vi "Network Command Engine.vi"(8 "error in (no error)":errorcluster, 11 "State Variables":T1={"TCP Refs"={"Connection List"=refnum, "listener ID"=refnum}, "Stop"=refnum, "Top VI"=refnum, "Parameters"={"Name"="", "PID Lookup"=variant, "DID Lookup"=variant, "Section Properties"={"CAN"={"Database File"=path "", "CAN Interface"=enum."CAN0", "Baud Rate"=0, "Diagnostic Protocol"=enum."GMLAN", "Transport Protocol"=enum."ISO TP - Normal Mode", "Transmit ID"=0, "Receive ID"=0, "Transmit Extension"=0, "Receive Extension"=0, "Receive UUDT ID"=0, "Enable Stream"=TRUE, "VW TP Channel ID"=0}, "DPIDs"=[], "DTC descriptor"={"DTC Byte Length"=2, "Status Byte Length"=1, "Add Data Byte Length"=1, "Byte Order"=enum."Motorola"}, "PIDs"=[], "DIDs"=[], "CPIDs"=[]}, "ChanRefs"={"ToVS.PIDs"={"Name"="", "Write to VS Engine FIFO"=refnum, "Pairs"={"Refs"=[], "Values"=[]}}, "ToVS.DIDs"={"Name"="", "Write to VS Engine FIFO"=refnum, "Pairs"={"Refs"=[], "Values"=[]}}, "ToVS.DTCs"={"Name"="", "Write to VS Engine FIFO"=refnum, "Pairs"={"Refs"=[], "Values"=[]}}, "ToVS.DTCCount"={"Name"="", "Write to VS Engine FIFO"=refnum, "Pairs"={"Refs"=[], "Values"=[]}}, "ToVS.Success"={"Name"="", "Write to VS Engine FIFO"=refnum, "Pairs"={"Refs"=[], "Values"=[]}}, "FromVS.CPIDs"={"Name"="", "Read from VS Engine FIFO"=refnum, "Pairs"={"Refs"=[], "Values"=[]}}, "Cmds"={"Name"="", "Write to VS Engine FIFO"=refnum, "Read from VS Engine FIFO"=refnum, "Pairs"={"Chan Refs"=[], "Prev. Values"=[]}}}, "CPID Lookup"=variant, "DPID Lookup"=variant}, "ADCS Connection"={"Diag CAN Handle"=0, "Transport Protocol"=enum."ISO TP - Normal Mode", "Receive Address Extension"=0, "Transmit Address Extension"=0, "Receive CAN Id"=0, "Transmit CAN Id"=0, "Diag CAN Queue"=refnum, "Log Frames ?"=FALSE, "My TP Address"=0, "Other TP Address"=0, "T1"=0, "T2"=0, "T3"=0, "T4"=0, "Tx SN"=0, "Block Size"=0, "Rx SN"=0, "VW TP Initialized?"=FALSE, "Tx block no"=0, "baud rate"=0, "Interface"="", "Channel Diag CAN Handle"=0, "UDP Connection ID"=refnum, "TCP Connection ID"=refnum, "Target IP Addr"=0, "Source Address"=0, "Target Address"=0, "Send Header NACK?"=FALSE, "DLL Handle"=0, "NAD"=0, "Time Stamp read first"=0.0, "Time Stamp read last"=0.0, "Time Stamp write first"=0.0, "Time Stamp write last"=0.0, "Time Stamp write"=0.0, "Time Stamp read"=0.0}, "XNET References"={"Database"="", "GMLAN DPID Session"="", "Cluster"=""}, "BufferedCmds"=refnum, "XNETEngine (GMLAN)"=refnum} {"Parameters"."ChanRefs"."Cmds"."Pairs"."Chan Refs" format="%.0x"; "Parameters"."ChanRefs"."ToVS.Success"."Pairs"."Refs" format="%.0x"; "Parameters"."ChanRefs"."ToVS.DTCCount"."Pairs"."Refs" format="%.0x"; "Parameters"."ChanRefs"."ToVS.DTCs"."Pairs"."Refs" format="%.0x"; "Parameters"."ChanRefs"."ToVS.PIDs"."Pairs"."Refs" format="%.0x"; "Parameters"."ChanRefs"."ToVS.DIDs"."Pairs"."Refs" format="%.0x"; "Parameters"."Section Properties"."CPIDs"."Signals"."Byte Order" items=["Little Endian", "Big Endian"]; "Parameters"."Section Properties"."CPIDs"."Signals"."Data Type" items=["Signed", "Unsigned", "IEEE Float"]; "Parameters"."Section Properties"."DIDs"."Signals"."Byte Order" items=["Little Endian", "Big Endian"]; "Parameters"."Section Properties"."DIDs"."Signals"."Data Type" items=["Signed", "Unsigned", "IEEE Float"]; "Parameters"."Section Properties"."CAN"."VW TP Channel ID" format="%.0x"; "Parameters"."Section Properties"."CAN"."Receive UUDT ID" format="%.0x"; "Parameters"."Section Properties"."CAN"."Receive Extension" format="%.0x"; "Parameters"."Section Properties"."CAN"."Transmit Extension" format="%.0x"; "Parameters"."Section Properties"."CAN"."Receive ID" format="%.0x"; "Parameters"."Section Properties"."CAN"."Transmit ID" format="%.0x"; "Parameters"."Section Properties"."PIDs"."Signals"."Byte Order" items=["Little Endian", "Big Endian"]; "Parameters"."Section Properties"."PIDs"."Signals"."Data Type" items=["Signed", "Unsigned", "IEEE Float"]}) -> (0 "error out":errorcluster)   [LabVIEW 2015, in "Diagnostics Addon Engine.lvlib"]
uses:
  Diagnostics Addon Engine.lvlib
  State Variables.ctl
  TCP Refs.ctl
  STM/STM Lookup Table Ref.ctl
  Stop FG/Stop Global Ref.ctl
  Main Configuration.ctl
  Section Properties.ctl
  Shared/CAN Configuration.ctl
  Shared/CAN Interface.ctl
  Shared/Diagnostic Protocols.ctl
  Shared/Transport Protocols.ctl
  Shared/DPID Parameters.ctl
  Shared/DPID Periodic Rate.ctl
  <vilib>/Automotive Diagnostic Command Set/Diagnostic Protocols.llb/DTC Descriptor.ctl
  Shared/DIDPID Parameters.ctl
  Shared/DIDPID Signal Parameters.ctl
  VS Data Channels.ctl
  Inline Async API/Controls/Write To VS Engine.ctl
  <vilib>/NI Veristand/Custom Device API/Data Reference.ctl
  Inline Async API/Controls/Read From VS Engine.ctl
  <vilib>/NI Veristand/Custom Device API/Block Data Reference.ctl
  Inline Async API/Controls/ReadWrite Data.ctl
  <vilib>/Automotive Diagnostic Command Set/Diagnostic Transport.llb/Diag Reference.ctl
  <vilib>/Automotive Diagnostic Command Set/Diagnostic Transport.llb/Transport Protocol Selector.ctl
  <vilib>/Automotive Diagnostic Command Set/Diagnostic Transport.llb/Diag CAN Frame Log.ctl
  XNET References.ctl
  <vilib>/NI/AMC/Message Queue.ctl
  <vilib>/NI/AMC/Message.ctl
  <vilib>/NI/Tools/Keyed Array/KeyedArray.ctl
  STM/Connection Manager/stm_TCPConnectionMethod.ctl
  Stop FG/Stop Global Commands.ctl
  STM/TCP/stm_TCP Read Options.ctl
  Shared/RequestResponse Data Cluster.ctl
  STM/TCP/stm_TCP Write Options.ctl
  STM/_SubVIs/stm_MetaDataElement.ctl
  <vilib>/NI/Tools/Keyed Array/Map String.vi
  <vilib>/NI/AMC/Create Single Message.vi
  <vilib>/NI/AMC/Update Message Routing Info.vi
  <vilib>/NI/AMC/Read Termination Message.vi
  <vilib>/NI/Tools/String/Get Case Matching.vi
  <vilib>/NI/AMC/Send Message.vi
  <vilib>/NI/AMC/Globals.vi
  Shared/GUID Lookup.vi
  Stop FG/Stop FG.lvlib
  Error Handling API/Error Handling API.lvlib
  Shared/Diagnostics Addon Shared.lvlib
  <vilib>/NI Veristand/Custom Device Tools/Custom Device Utility Library/Custom Device Utility Library.lvlib
  <vilib>/NI/Tools/Keyed Array/Tools_KeyedArray.lvlib
  <vilib>/NI/AMC/AMC.lvlib
  <vilib>/NI Veristand/Custom Device API/Custom Device API.lvlib
  <vilib>/addons/Automotive Diagnostic Command Set/NI_Automotive Diagnostic Command Set.lvlib
  Inline Async API/Inline Async API.lvlib
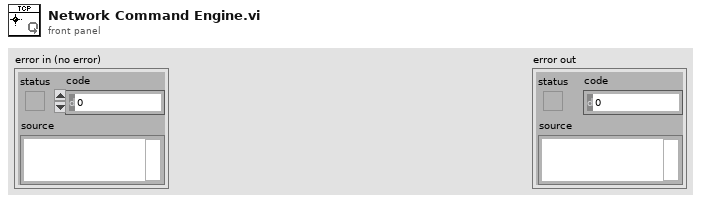
[diagram p1: front panel]
types:
  T1 = typedef "Diagnostics Addon Engine.lvlib/State Variables.ctl" = cluster{"TCP Refs":T2, "Stop":T4, "Top VI":refnum<vi>, "Parameters":T5, "ADCS Connection":T22, "XNET References":T24, "BufferedCmds":T25, "XNETEngine (GMLAN)":T25}
  T2 = typedef "Diagnostics Addon Engine.lvlib/TCP Refs.ctl" = cluster{"Connection List":T3, "listener ID":refnum<k5>}
  T3 = typedef "Diagnostics Addon Engine.lvlib/STM Lookup Table Ref.ctl" = refnum<vi>
  T4 = typedef "Diagnostics Addon Engine.lvlib/Stop FG.lvlib/Stop Global Ref.ctl" = refnum<vi>
  T5 = typedef "Diagnostics Addon Engine.lvlib/Main Configuration.ctl" = cluster{"Name":string, "PID Lookup":variant, "DID Lookup":variant, "Section Properties":T6, "ChanRefs":T16, "CPID Lookup":variant, "DPID Lookup":variant}
  T6 = typedef "Diagnostics Addon Engine.lvlib/Section Properties.ctl" = cluster{"CAN":T7, "DPIDs":T11[], "DTC descriptor":T13, "PIDs":T14[], "DIDs":T14[], "CPIDs":T14[]}
  T7 = typedef "Diagnostics Addon Shared.lvlib/CAN Configuration.ctl" = cluster{"Database File":path, "CAN Interface":T8, "Baud Rate":u32, "Diagnostic Protocol":T9, "Transport Protocol":T10, "Transmit ID":u32, "Receive ID":u32, "Transmit Extension":u8, "Receive Extension":u8, "Receive UUDT ID":u32, "Enable Stream":bool, "VW TP Channel ID":u32}
  T8 = typedef "Diagnostics Addon Shared.lvlib/CAN Interface.ctl" = enum16{"CAN0", "CAN1", "CAN2", "CAN3", "CAN4", "CAN5", "CAN6", "CAN7", "CAN8", "CAN9", "CAN10", "CAN11", "CAN12", "CAN13", "CAN14", "CAN15", "CAN16", "CAN17", "CAN18", "CAN19", "CAN20", "CAN21", "CAN22", "CAN23", "CAN24", "CAN25", "CAN26", "CAN27", "CAN28", "CAN29", "CAN30", "CAN31", "CAN32", "CAN33", "CAN34", "CAN35", "CAN36", "CAN37", "CAN38", "CAN39", "CAN40", "CAN41", "CAN42", "CAN43", "CAN44", "CAN45", "CAN46", "CAN47", "CAN48", "CAN49", "CAN50", "CAN51", "CAN52", "CAN53", "CAN54", "CAN55", "CAN56", "CAN57", "CAN58", "CAN59", "CAN60", "CAN61", "CAN62", "CAN63", "CAN 256 (Virtual)", "CAN 257 (Virtual)"}
  T9 = typedef "Diagnostics Addon Shared.lvlib/Diagnostic Protocols.ctl" = enum16{"GMLAN", "KWP-2000", "UDS"}
  T10 = typedef "Diagnostics Addon Shared.lvlib/Transport Protocols.ctl" = enum16{"ISO TP - Normal Mode", "ISO TP - Mixed Mode", "VW TP 2.0", "Diagnostics on IP"}
  T11 = typedef "Diagnostics Addon Shared.lvlib/DPID Parameters.ctl" = cluster{"DPID ID":u8, "Speed":T12, "PIDs":u16[]}
  T12 = typedef "Diagnostics Addon Shared.lvlib/DPID Periodic Rate.ctl" = enum16{"Slow", "Medium", "Fast"}
  T13 = typedef "DTC Descriptor.ctl" = cluster{"DTC Byte Length":i32, "Status Byte Length":i32, "Add Data Byte Length":i32, "Byte Order":enum16{"Motorola", "Intel"}}
  T14 = typedef "Diagnostics Addon Shared.lvlib/DIDPID Parameters.ctl" = cluster{"Name":string, "Description":string, "ID":u16, "Signals":T15[]}
  T15 = typedef "Diagnostics Addon Shared.lvlib/DIDPID Signal Parameters.ctl" = cluster{"Start Bit":u8, "Length":u8, "Scaling Factor":dbl, "Scaling Offset":dbl, "Minimum":dbl, "Maximum":dbl, "Data Type":u32, "Byte Order":u32, "Default Value":dbl, "Name":string, "Units":string, "Description":string}
  T16 = typedef "Diagnostics Addon Engine.lvlib/VS Data Channels.ctl" = cluster{"ToVS.PIDs":T17, "ToVS.DIDs":T17, "ToVS.DTCs":T17, "ToVS.DTCCount":T17, "ToVS.Success":T17, "FromVS.CPIDs":T19, "Cmds":T21}
  T17 = typedef "Diagnostics Addon Engine.lvlib/Inline Async API.lvlib/Write To VS Engine.ctl" = cluster{"Name":string, "Write to VS Engine FIFO":refnum<k33>, "Pairs":cluster{"Refs":T18[], "Values":dbl[]}}
  T18 = typedef "Custom Device API.lvlib/Data Reference.ctl" = i32
  T19 = typedef "Diagnostics Addon Engine.lvlib/Inline Async API.lvlib/Read From VS Engine.ctl" = cluster{"Name":string, "Read from VS Engine FIFO":refnum<k33>, "Pairs":cluster{"Refs":T20[], "Values":dbl[]}}
  T20 = typedef "Custom Device API.lvlib/Block Data Reference.ctl" = cluster{"Data Reference":T18, "Offset":u64, "Length":u64}
  T21 = typedef "Diagnostics Addon Engine.lvlib/Inline Async API.lvlib/ReadWrite Data.ctl" = cluster{"Name":string, "Write to VS Engine FIFO":refnum<k33>, "Read from VS Engine FIFO":refnum<k33>, "Pairs":cluster{"Chan Refs":T18[], "Prev. Values":dbl[]}}
  T22 = typedef "NI_Automotive Diagnostic Command Set.lvlib/Diag Reference.ctl" = cluster{"Diag CAN Handle":u32, "Transport Protocol":T23, "Receive Address Extension":u8, "Transmit Address Extension":u8, "Receive CAN Id":u32, "Transmit CAN Id":u32, "Diag CAN Queue":refnum<queue>, "Log Frames ?":bool, "My TP Address":u8, "Other TP Address":u8, "T1":u16, "T2":u16, "T3":u16, "T4":u16, "Tx SN":u8, "Block Size":u8, "Rx SN":u8, "VW TP Initialized?":bool, "Tx block no":u8, "baud rate":u32, "Interface":string, "Channel Diag CAN Handle":u32, "UDP Connection ID":refnum<k16>, "TCP Connection ID":refnum<k5>, "Target IP Addr":u32, "Source Address":u16, "Target Address":u16, "Send Header NACK?":bool, "DLL Handle":u32, "NAD":u8, "Time Stamp read first":dbl, "Time Stamp read last":dbl, "Time Stamp write first":dbl, "Time Stamp write last":dbl, "Time Stamp write":dbl, "Time Stamp read":dbl}
  T23 = typedef "NI_Automotive Diagnostic Command Set.lvlib/Transport Protocol Selector.ctl" = enum16{"ISO TP - Normal Mode", "ISO TP - Mixed Mode", "VW TP 2.0", "Diagnostics on IP", "ISO TP LIN"}
  T24 = typedef "Diagnostics Addon Engine.lvlib/XNET References.ctl" = cluster{"Database":refnum<k21>, "GMLAN DPID Session":refnum<k21>, "Cluster":refnum<k21>}
  T25 = typedef "AMC.lvlib/Message Queue.ctl" = refnum<queue>
  T26 = typedef "Diagnostics Addon Engine.lvlib/Stop FG.lvlib/Stop Global Commands.ctl" = enum16{"Write", "Read", "Reset"}
  T27 = typedef "Diagnostics Addon Engine.lvlib/stm_TCPConnectionMethod.ctl" = enum16{"Initialize", "Add Connection", "Set Properties", "Get Connection(s)", "Remove Connection", "Remove All Connections", "Get Connection Count"}
  T28 = typedef "Diagnostics Addon Engine.lvlib/stm_TCP Read Options.ctl" = cluster{"Ignore Timeout Error":bool, "timeout ms (1000)":i32}
  T29 = typedef "Diagnostics Addon Engine.lvlib/stm_TCP Write Options.ctl" = cluster{"Ignore Timeout Error":bool, "timeout ms (1000)":i32}
  T30 = typedef "Diagnostics Addon Shared.lvlib/RequestResponse Data Cluster.ctl" = cluster{"Timeout":i32, "data":string}
  T31 = typedef "Diagnostics Addon Engine.lvlib/stm_MetaDataElement.ctl" = string
  T32 = typedef "Diagnostics Addon Engine.lvlib/stm_TCP Connection Info.ctl" = cluster{"connection ID":refnum<k5>, "Meta data":T31[]}
  T33 = typedef "Tools_KeyedArray.lvlib/KeyedArray.ctl" = cluster{"keys":string[], "values":string[]}
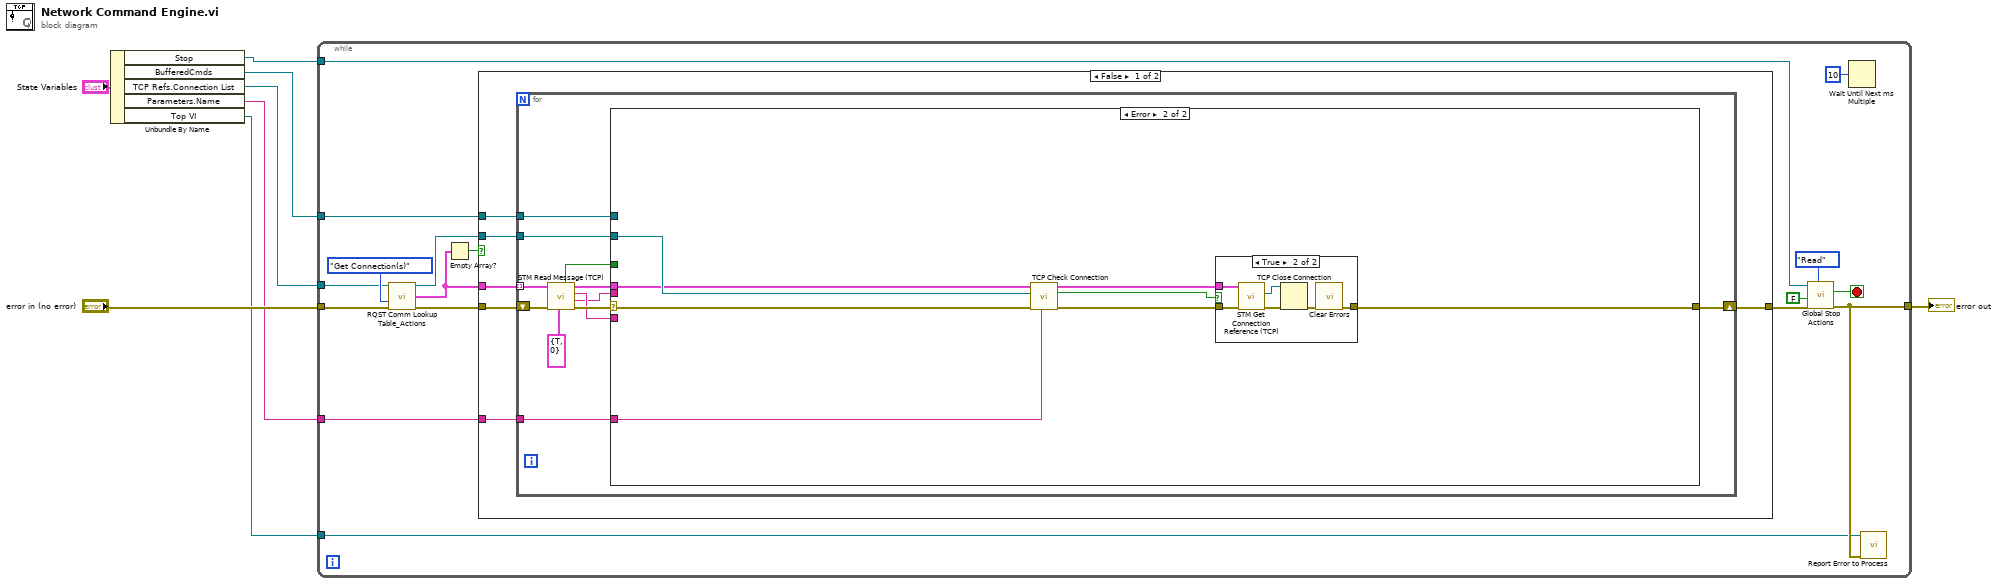
[diagram p0: block diagram]
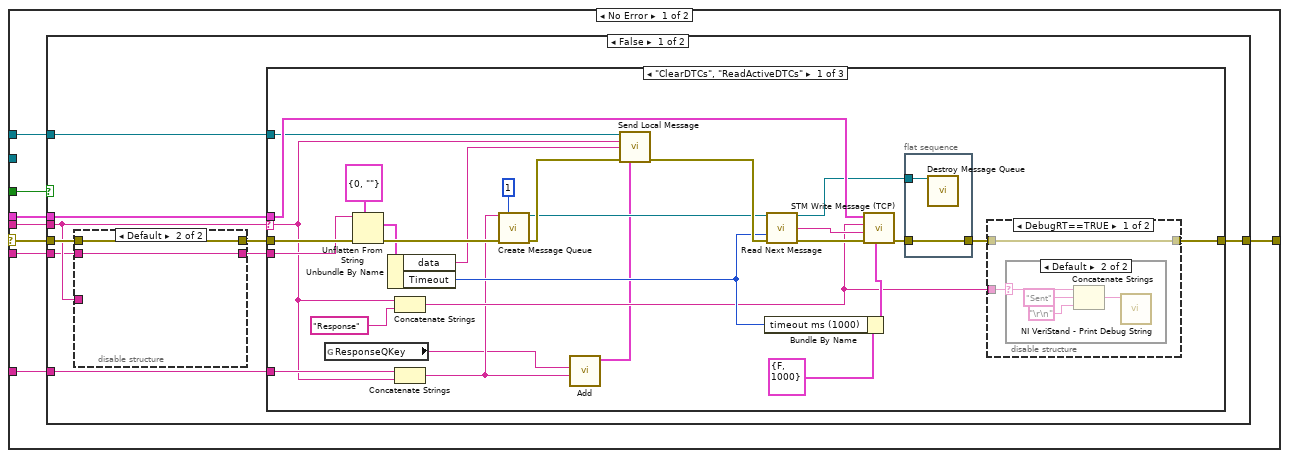
[diagram p2: hidden frame]
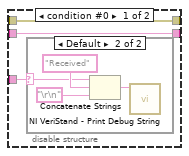
[diagram p3: hidden frame]
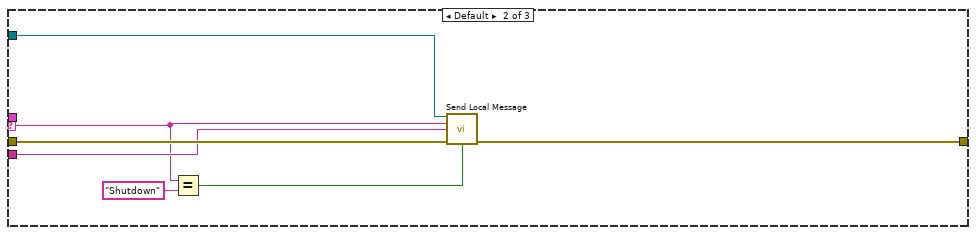
[diagram p7: hidden frame]
diagram:
  n1 = Unbundle By Name("State Variables") -> ("Stop"=w8:T4, "BufferedCmds"=w1:T25, "TCP Refs.Connection List"=w6:T3, "Parameters.Name"=w2:string, "Top VI"=w3:refnum<vi>)
  n2 = while {
    tunnel: "error in (no error)" -> [w21]
    tunnel: [w15] -> w4
    tunnel: w6 -> [w14]
    tunnel: w8 -> [w13]
    tunnel: w2 -> [w12]
    tunnel: w3 -> [w10]
    tunnel: w1 -> [w9]
    stop <- w16 stop-if-true
    n3 = call "RQST Comm Lookup Table_Actions.vi"("ref in"=w14, "Method"=stm_TCPConnectionMethod."Get Connection(s)", "error in (no error)"=w21) -> ("ref out"=w19:T3, "All Connections"=w22:T32[], "error out"=w20:errorcluster)  [unwired: 6 in, 4 out]
    n4 = Empty Array?(array=w22) -> (empty?=w23:bool)
    n5 = case shown="False" w23 {
      tunnel: w22 -> [w31 _]
      tunnel: w20 -> [w27 w131]
      tunnel: w19 -> [w30 _]
      tunnel: [w29 w131] -> w17
      tunnel: w12 -> [w28 _]
      tunnel: w9 -> [w26 _]
      frame False {
        n6 = for {
          tunnel: w31 -> [w38] mode=indexing
          tunnel: w30 -> [w43]
          shift-right: [w42] -> w29
          shift-left: w27 -> [w40]
          tunnel: w28 -> [w41]
          tunnel: w26 -> [w32]
          n7 = call "STM Read Message (TCP).vi"("Options"=T28 {"Ignore Timeout Error"=TRUE, "timeout ms (1000)"=0}, "error in"=w40, "Connection Info"=w38) -> ("error out"=w39:errorcluster, "Name"=w34:T31, "data string"=w35:string, "Connection Info"=w37:T32, "Timed Out?"=w33:bool)  [unwired: 3 in, 1 out]
          n8 = case shown="Error" w39 {
            selector: w39 -> [w51 w118]
            tunnel: w43 -> [_ w120]
            tunnel: w37 -> [w44 w119]
            tunnel: [w50 w117] -> w42
            tunnel: w41 -> [w45 w116]
            tunnel: w35 -> [w49 _]
            tunnel: w34 -> [w48 _]
            tunnel: w33 -> [w47 _]
            tunnel: w32 -> [w46 _]
            frame No Error {
              n9 = case shown="False" w47 {
                tunnel: w51 -> [w56 w115]
                tunnel: [w60 w115] -> w50
                tunnel: w49 -> [w52 _]
                tunnel: w48 -> [w54 _]
                tunnel: w46 -> [w59 _]
                tunnel: w45 -> [w58 _]
                tunnel: w44 -> [w57 _]
                frame False {
                  n10 = disable-structure shown="Default" {
                    disable-tunnel: w54 -> [w63 _]
                    disable-tunnel: [w62 w69] -> w55
                    disable-tunnel: w56 -> [w62 w69]
                    disable-tunnel: [w61 w68] -> w53
                    disable-tunnel: w52 -> [w61 w68]
                    frame condition #0 {
                      n11 = case shown="Default" w63 {
                        selector: w63 -> [_ w65]
                        frame "" {
                        }
                        frame Default {
                          n12 = Concatenate Strings(w65, "Received" ("string"), "\r\n") -> (w67:string)
                          n13 = call <vilib>:"NI VeriStand - Print Debug String.vi"("Message"=w67) -> ()  [unwired: 10 in, 1 out]
                        }
                      }
                    }
                    frame condition #1 (active) {
                    }
                  }
                  n14 = case shown="\"ClearDTCs\", \"ReadActiveDTCs\"" w54 {
                    selector: w54 -> [w86 w108 _]
                    tunnel: w55 -> [w93 w113 w114]
                    tunnel: [w76 w112 w114] -> w60
                    tunnel: w53 -> [w89 w111 _]
                    tunnel: w59 -> [w71 w107 _]
                    tunnel: w58 -> [w97 _ _]
                    tunnel: w57 -> [w84 _ _]
                    frame "ClearDTCs", "ReadActiveDTCs" {
                      n15 = global read "GUID Lookup.vi" "ResponseQKey"() -> (w72:string)
                      n16 = Unflatten From String(type=T30 {"Timeout"=0, "data"=""}, binary string=w89, error in (no error)=w93) -> (value=w90:T30, error out=w92:errorcluster)  [unwired: 2 in, 1 out]
                      n17 = Unbundle By Name(w90) -> ("data"=w88:string, "Timeout"=w81:i32)
                      n18 = Concatenate Strings(w86, "Response" ("string")) -> (w78:string)
                      n19 = Concatenate Strings(w97, w86) -> (w75:string)
                      n20 = call <vilib>:"Create Message Queue.vi"("message queue name"=w75, "max queue size (-1, unlimited)"=1, "error in"=w92) -> ("message queue out"=w94:T25, "error out"=w96:errorcluster)  [unwired: 11 in]
                      n21 = call <vilib>:"Add.vi"("value"=w75, "key"=w72) -> ("array out"=w74:T33)  [unwired: 3 in, 2 out]
                      n22 = call <vilib>:"Send Local Message.vi"("message queue in"=w71, "message name"=w86, "message value"=w88, "error in"=w96, "message attributes"=w74) -> ("error out"=w95:errorcluster)  [unwired: 8 in, 2 out]
                      n23 = Bundle By Name(cluster=T29 {"Ignore Timeout Error"=FALSE, "timeout ms (1000)"=1000} ("Options"), "timeout ms (1000)"=w81) -> (w82:T29)
                      n24 = call <vilib>:"Read Next Message.vi"("message queue in"=w94, "timeout (1 ms)"=w81, "error in"=w95) -> ("message queue out"=w80:T25, "message value"=w85:string, "error out"=w87:errorcluster)  [unwired: 5 in, 5 out]
                      n25 = call "STM Write Message (TCP).vi"("Options"=w82, "error in (no error)"=w87, "Data"=w85, "Name"=w78, "Connection Info"=w84) -> ("error out"=w79:errorcluster)  [unwired: 5 in, 1 out]
                      n26 = flat-sequence {
                        tunnel: w80 -> [w106]
                        tunnel: w79 -> [w105]
                        tunnel: [w105] -> w77
                        frame #0 {
                          n27 = call <vilib>:"Destroy Message Queue.vi"("message queue in"=w106) -> ()  [unwired: 12 in, 3 out]
                        }
                      }
                      n28 = disable-structure shown="DebugRT==TRUE" {
                        disable-tunnel: w78 -> [w99 _]
                        disable-tunnel: [w98 w104] -> w76
                        disable-tunnel: w77 -> [w98 w104]
                        frame condition #0 {
                          n29 = case shown="Default" w99 {
                            selector: w99 -> [_ w101]
                            frame "" {
                            }
                            frame Default {
                              n30 = Concatenate Strings(w101, "Sent" ("string"), "\r\n") -> (w103:string)
                              n31 = call <vilib>:"NI VeriStand - Print Debug String.vi"("Message"=w103) -> ()  [unwired: 10 in, 1 out]
                            }
                          }
                        }
                        frame condition #1 (active) {
                        }
                      }
                    }
                    frame Default {
                      n32 = Equal?(x=w108, y=T31 "Shutdown" ("x")) -> (x = y?=w110:bool)
                      n33 = call <vilib>:"Send Local Message.vi"("message queue in"=w107, "message name"=w108, "message value"=w111, "error in"=w113, "priority message (F)"=w110) -> ("error out"=w112:errorcluster)  [unwired: 8 in, 2 out]
                    }
                    frame "" {
                    }
                  }
                }
                frame True {
                }
              }
            }
            frame Error {
              n34 = call "TCP Check Connection.vi"("Name"=w116, "error in (no error)"=w118, "ref in"=w120, "Connection In"=w119) -> ("error out"=w123:errorcluster, "Disconnected"=w121:bool, "Connection In"=w122:T32)  [unwired: 5 in]
              n35 = case shown="True" w121 {
                tunnel: [w124 w127] -> w117
                tunnel: w123 -> [w124 w130]
                tunnel: w122 -> [_ w125]
                frame False {
                }
                frame True {
                  n36 = call "STM Get Connection Reference (TCP).vi"("error in"=w130, "Connection Info"=w125) -> ("error out"=w129:errorcluster, "connection ID out"=w128:refnum<k5>)  [unwired: 7 in, 1 out]
                  n37 = TCP Close Connection(connection ID=w128, error in (no error)=w129) -> (error out=w126:errorcluster)  [unwired: 1 in, 1 out]
                  n38 = call <vilib>:"Clear Errors.vi"("error in (no error)"=w126) -> ("error out"=w127:errorcluster)  [unwired: 5 in, 1 out]
                }
              }
            }
          }
        }
      }
      frame True {
      }
    }
    n39 = call "Global Stop Actions.vi"("Command"=Stop_Global_Commands."Read", "error in (no error)"=w17, "Stop on Error?"=FALSE, "vi reference"=w13) -> ("error out"=w15:errorcluster, "Latched Stop"=w16:bool)  [unwired: 5 in, 1 out]
    n40 = Wait Until Next ms Multiple(millisecond multiple=u32 10 ("STM Update Rate")) -> ()  [unwired: 1 out]
    n41 = call "Report Error to Process.vi"("Error"=w15, "This VI"=w10) -> ()  [unwired: 10 in]
  }
  "error out" <- w4
